vi "Parse Frame Config Data (subVI).vi"(8 "error in (no error)":errorcluster, 10 "CSV Raw Data":string[][](array[string]), 11 "Config Parser SPI_3W in":refnum<class "Config Parser SPI_3W.lvclass">) -> (0 "error out":errorcluster, 1 "Pattern Name out":string, 2 "Config Data out":string[](array[string]), 3 "Config Parser SPI_3W out":refnum<class "Config Parser SPI_3W.lvclass">)   [LabVIEW 2018, in "Config Parser SPI_3W.lvlib" / "Config Parser SPI_3W.lvclass"]
uses:
  Config Parser SPI_3W.lvclass
  Ctls/Frame Data - SPI_3W.ctl
  Ctls/RW Options.ctl
  Interfaces/File Parser Interface.lvlibp/Interfaces/File Parser Interface/File Parser Interface.lvclass
  C:/P4 Workspace/PC Client/Solutions/5g_eap/trunk/1.0/HiSi5GmmWave/Pattern_Gen_Tool/Interfaces/File Parser Interface.lvlibp/Interfaces/File Parser Interface/File Parser Interface.lvclass
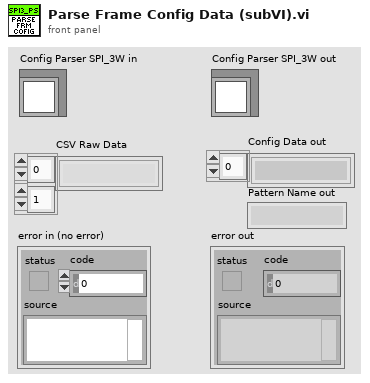
[diagram p1: front panel]
types:
  T1 = typedef "Frame Data - SPI_3W.ctl" = cluster{"Pattern Name":string, "Data":u16, "Addr":u16, "OpCode":string[], "R/W?":T2}
  T2 = typedef "RW Options.ctl" = enum16{"Read", "Write", "R/W"}
  T3 = typedef "File Parser Interface.lvlibp/RW Options.ctl" = enum16{"Read", "Write", "R/W"}
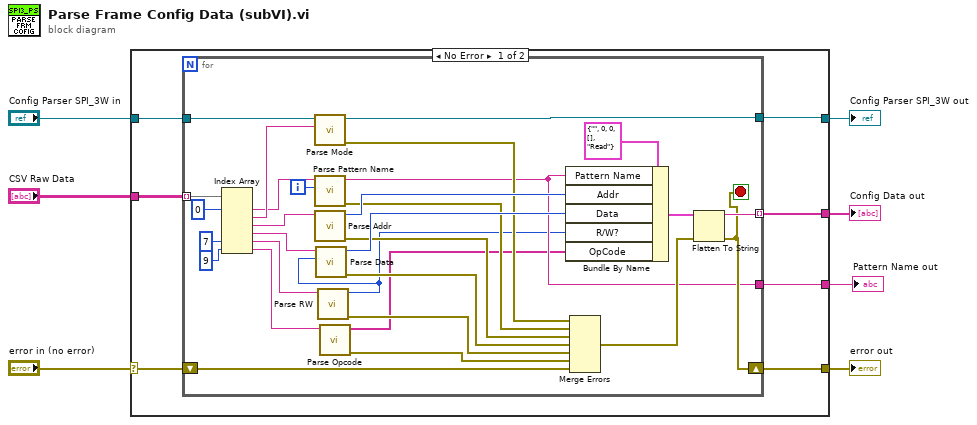
[diagram p0: block diagram]
diagram:
  n1 = case shown="No Error" "error in (no error)" {
    selector: "error in (no error)" -> [w14 w46]
    tunnel: [w13 w46] -> w6
    tunnel: [w10 w45] -> w4
    tunnel: "Config Parser SPI_3W in" -> [w11 w45]
    tunnel: "CSV Raw Data" -> [w12 _]
    tunnel: [w9 _] -> w2
    tunnel: [w8 _] -> w1
    frame No Error {
      n2 = for {
        shift-right: [w30] -> w13
        shift-left: w14 -> [w36]
        tunnel: w12 -> [w44] mode=indexing
        tunnel: w11 -> [w28]
        tunnel: [w27] -> w10
        tunnel: [w31] -> w9 mode=indexing
        tunnel: [w22] -> w8
        i -> [w23]
        stop <- w30 stop-if-true
        n3 = Index Array(array=w44, index #1=0 ("index"), index #5=7 ("index"), index #6=9 ("index")) -> (element #1=w24:string, element #2=w25:string, element #3=w40:string, element #4=w39:string, element #5=w20:string, element #6=w17:string)  [unwired: 3 in]
        n4 = call "Parse Mode.vi"("Protocol Mode in"=w25, "File Parser Interface in"=w28) -> ("error out"=w26:errorcluster, "File Parser Interface Out"=w27:refnum<class "Config Parser SPI_3W.lvclass">)  [unwired: 8 in]
        n5 = call "Parse Pattern Name.vi"("Index"=w23, "Pattern Name"=w24) -> ("error out"=w21:errorcluster, "Pattern Name out"=w22:string)  [unwired: 8 in]
        n6 = call "Parse Addr.vi"("Addr in"=w40) -> ("error out"=w34:errorcluster, "Addr out"=w38:u16)  [unwired: 9 in]
        n7 = call "Parse RW.vi"("R/W mode in"=w20) -> ("error out"=w19:errorcluster, "R/W?"=w18:T3)  [unwired: 9 in]
        n8 = call "Parse Data.vi"("R/W?"=w18, "Data in"=w39) -> ("error out"=w35:errorcluster, "Data out"=w37:u16)  [unwired: 8 in]
        n9 = call "Parse Opcode.vi"("Opcode"=w17) -> ("Error out"=w15:errorcluster, "Opcode Array"=w16:string[])  [unwired: 9 in]
        n10 = Bundle By Name(cluster=T1 {"Pattern Name"="", "Data"=0, "Addr"=0, "OpCode"=[], "R/W?"=enum."Read"} ("FRM Data"), "Pattern Name"=w22, "Addr"=w38, "Data"=w37, "R/W?"=w18, "OpCode"=w16) -> (w33:T1)
        n11 = Merge Errors(w26, w21, w34, w35, w19, w15, w36) -> (w32:errorcluster)
        n12 = Flatten To String(anything=w33, error in (no error)=w32) -> (data string=w31:string, error out=w30:errorcluster)  [unwired: 2 in, 1 out]
      }
    }
    frame Error {
    }
  }
  "error out" <- w6
  "Config Parser SPI_3W out" <- w4
  "Config Data out" <- w2
  "Pattern Name out" <- w1
